vi "DoubleWordToFloat.vi"(10 "register 2":u16, 11 "register":u16) -> (3 "Setpoint":sgl)   [LabVIEW 2018, in "Pid.lvlib"]
uses:
  Pid.lvlib
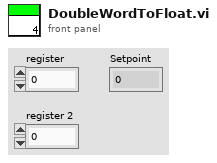
[diagram p1: front panel]
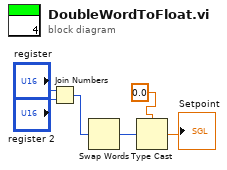
[diagram p0: block diagram]
diagram:
  n1 = Join Numbers(hi="register", lo="register 2") -> ((hi.lo)=w6:u32)
  n2 = Swap Words(1:w6) -> (0:w5:u32)
  n3 = Type Cast(type=sgl 0.0 ("Setpoint"), x=w5) -> (*(type *) &x=→"Setpoint":sgl)
